vi "Run (WaveIO).vi"(8 "error in (no error)":errorcluster, 11 "Audio Output Queue":refnum<queue>) -> (0 "error out":errorcluster)   [LabVIEW 2018, in "Audio Output.lvlib"]
doc: "The main audio output loop.\n\n<b>Priority:</b> Time Critical\n<b>Execution System:</b> Instrument I/O"
uses:
  Audio Output.lvlib
  Audio Output Queue Type.ctl
  State.ctl
  Messaging/Message Cluster.ctl
  Audio Output Config.ctl
  Audio Output Info.ctl
  external/waveio_108/WaveIO.llb/SoundHandle.ctl
  Globals/Debug.vi
  Messaging/Messaging.lvlib
  <vilib>/ptbypt/NI_PtbyPt.lvlib
  Globals/Globals.lvlib
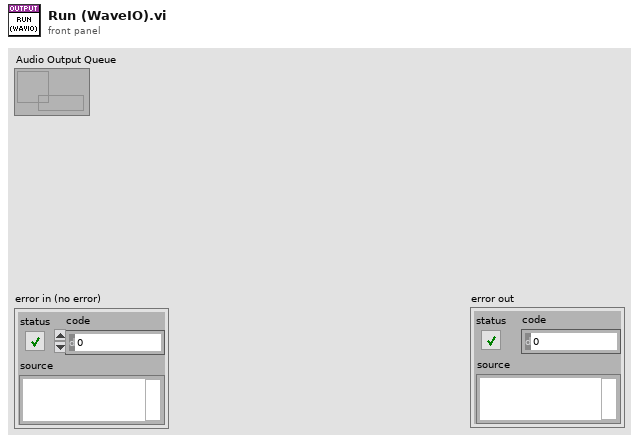
[diagram p1: front panel]
types:
  T1 = typedef "Audio Output.lvlib/Audio Output Config.ctl" = cluster{"Master":T2, "Headphones":T2}
  T2 = typedef "Audio Output.lvlib/Audio Output Info.ctl" = cluster{"Enable":bool, "Output ID":i32}
  T3 = typedef "Messaging.lvlib/Message Cluster.ctl" = cluster{"Event":string, "Source":string, "Target":string, "Data":variant}
  T4 = typedef "Audio Output.lvlib/State.ctl" = enum16{"Init", "Configure", "Output", "Error", "Shutdown"}
  T5 = typedef "SoundHandle.ctl" = cluster{"DeviceID":u16, "Samples/buf":u32, "Sampl rate":u32, "Bits/sample":u16, "Channels":u8, "Opened":bool}
  T6 = cluster{"# buffers":i32, "Buffer size":i32, "unit (ms)":enum16{"time (ms)", "Samples"}}
  T7 = typedef "Audio Output.lvlib/Audio Output Queue Type.ctl" = cluster{"Master":waveform(i16)[], "Headphones":waveform(i16)[], "Start Time":dbl}
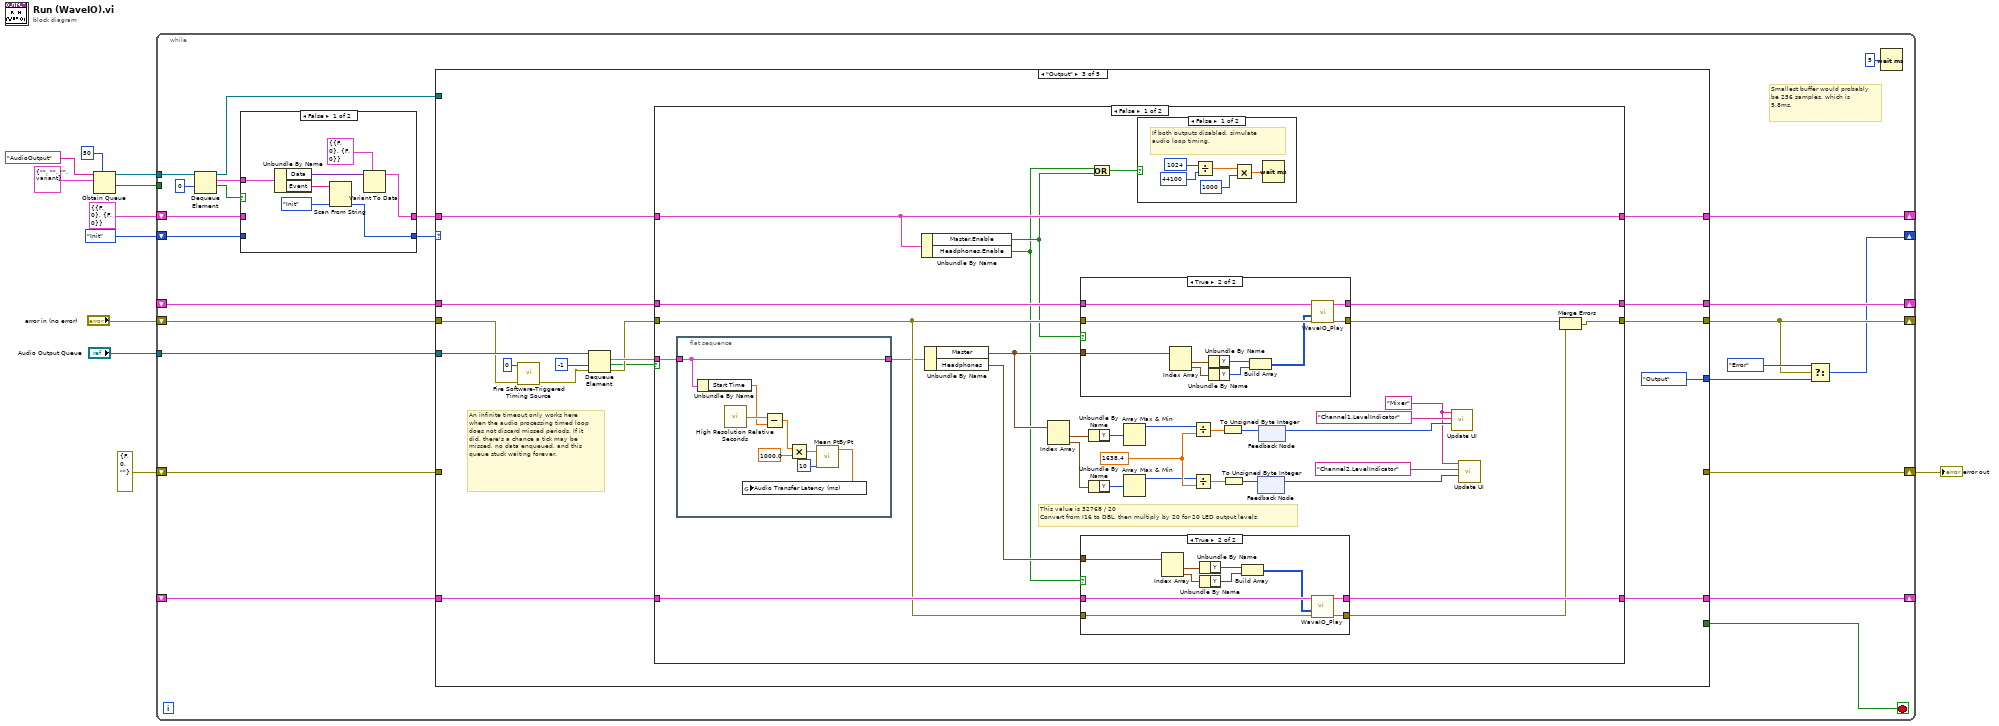
[diagram p0: block diagram]
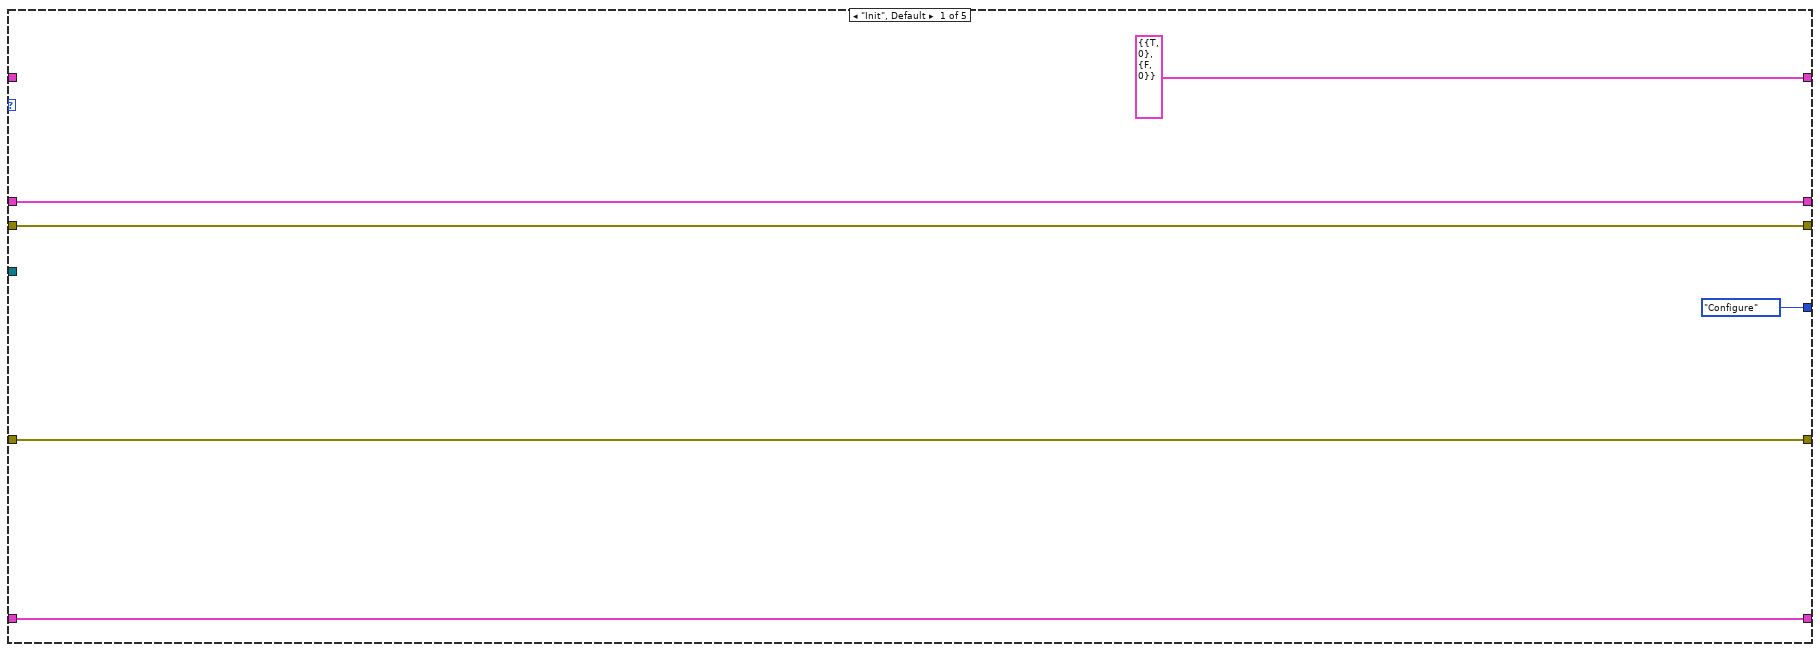
[diagram p3: hidden frame]
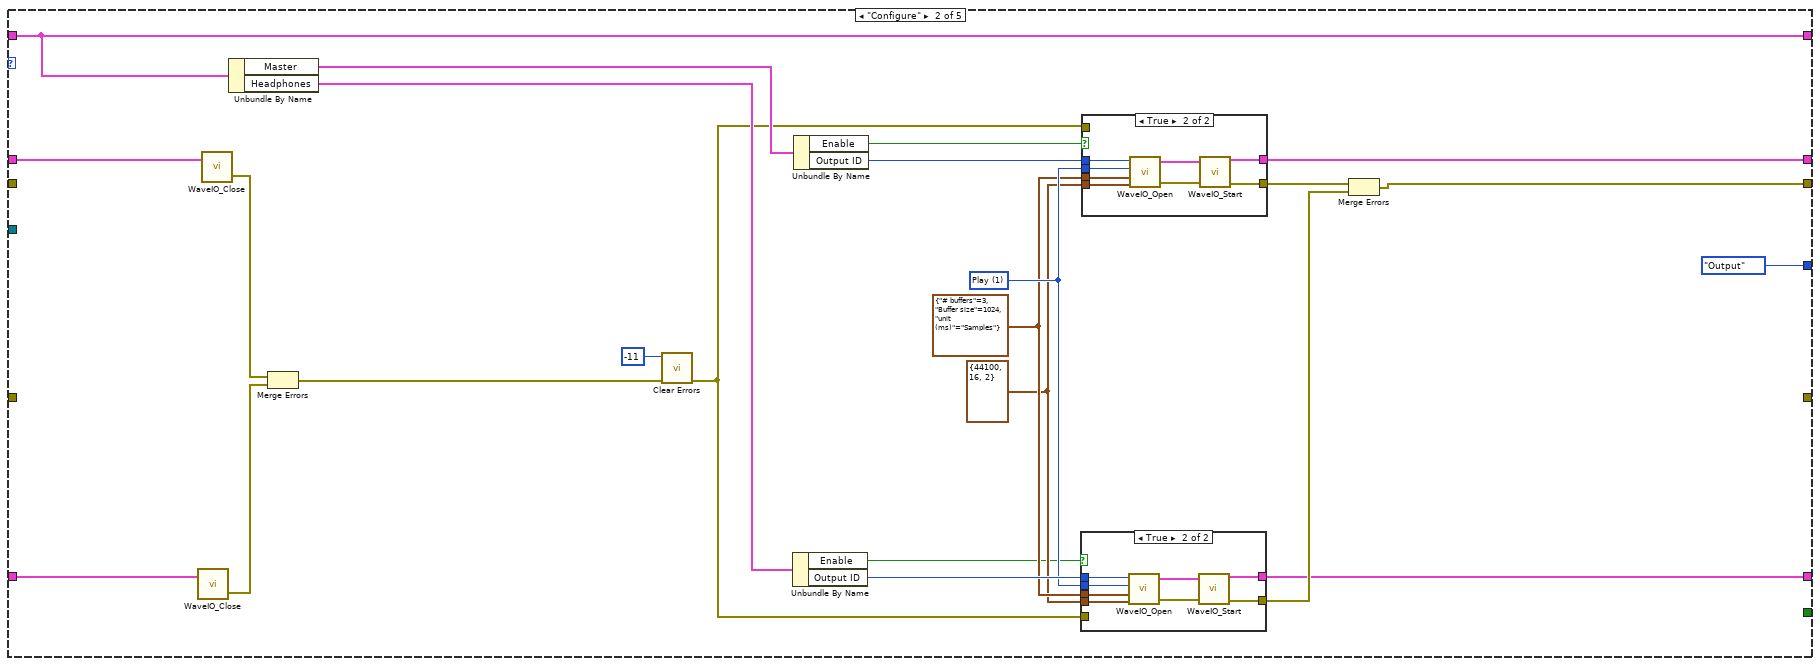
[diagram p4: hidden frame]
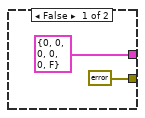
[diagram p5: hidden frame]
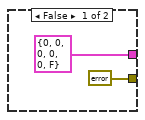
[diagram p6: hidden frame]
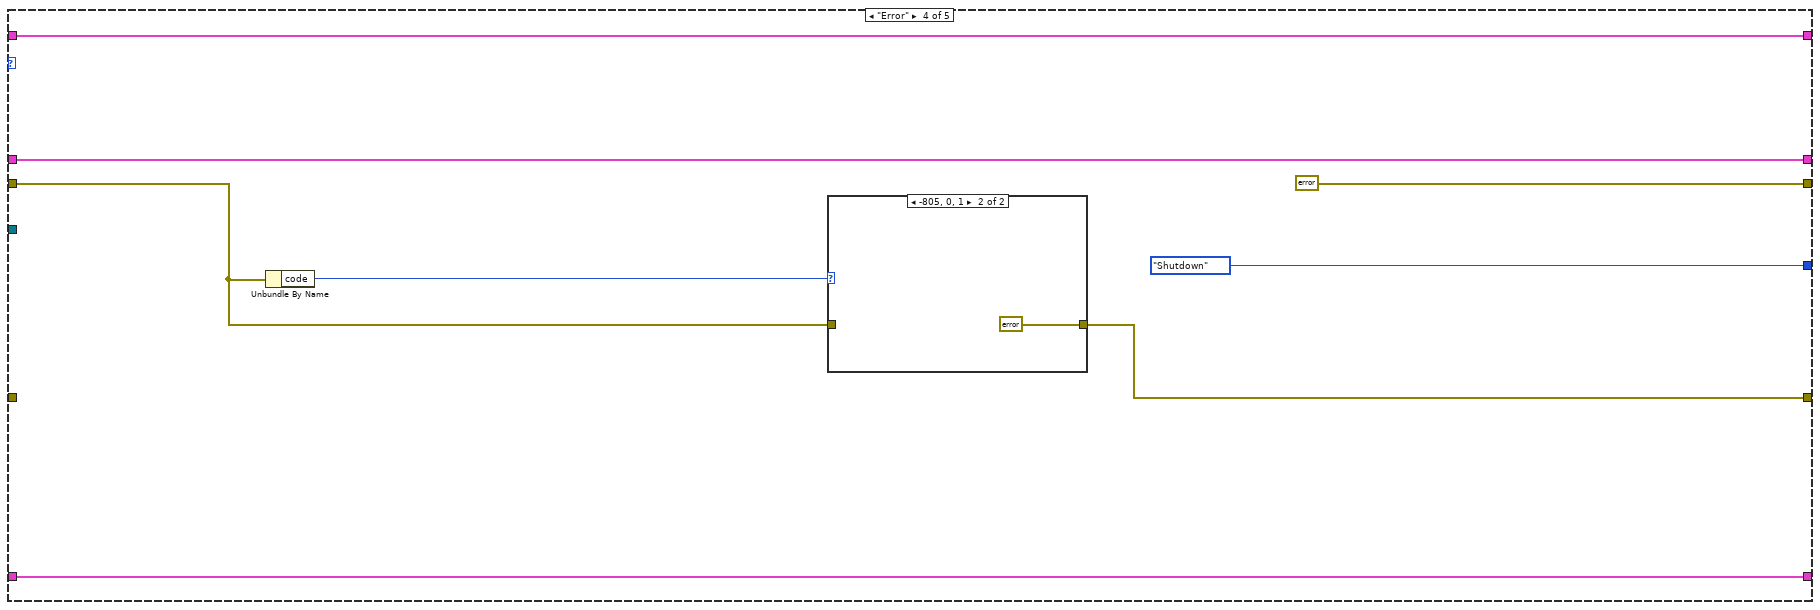
[diagram p11: hidden frame]
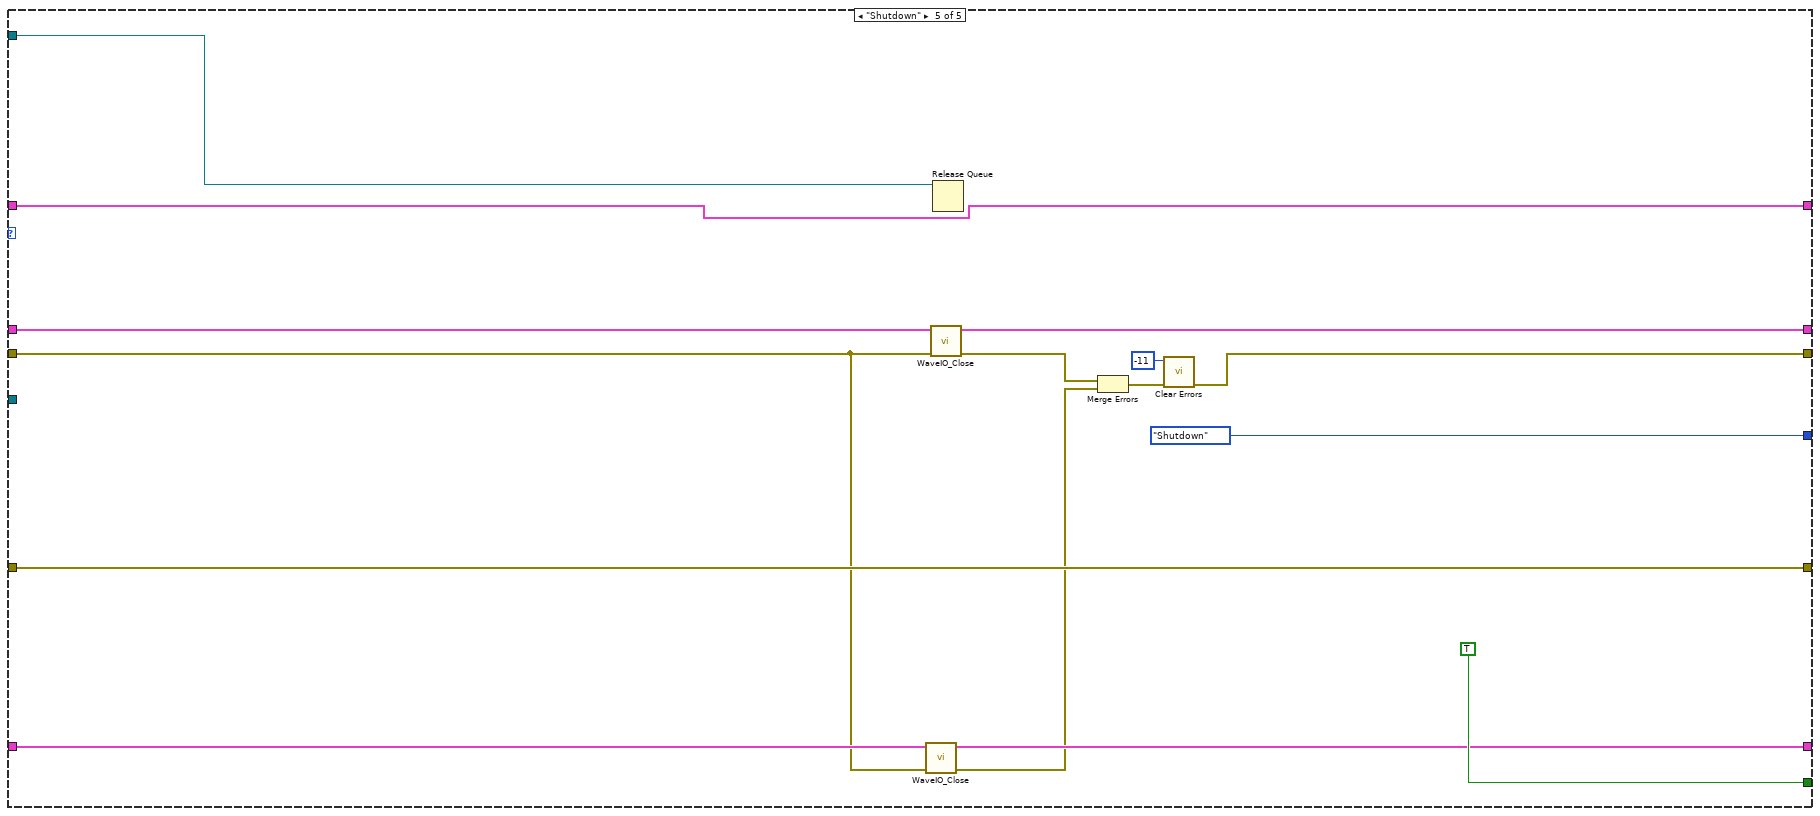
[diagram p13: hidden frame]
diagram:
  n1 = Obtain Queue(max queue size (-1, unlimited)=50, name (unnamed)="AudioOutput", element data type=T3 {"Event"="", "Source"="", "Target"="", "Data"=variant} ("Message")) -> (queue out=w4:refnum<queue>, created new?=w3:bool)  [unwired: 2 in, 1 out]
  n2 = while {
    shift-right: [w30] -> _
    shift-left: State."Init" ("State") -> [w19]
    shift-right: [w35] -> _
    shift-left: _ -> [w34]
    shift-right: [w31] -> _
    shift-left: "error in (no error)" -> [w29]
    tunnel: "Audio Output Queue" -> [w27]
    shift-right: [w26] -> w9
    shift-left: errorcluster {"status"=FALSE, "code"=0, "source"=""} ("error out") -> [w25]
    shift-right: [w24] -> _
    shift-left: _ -> [w23]
    tunnel: w4 -> [w21]
    shift-right: [w13] -> _
    shift-left: T1 {"Master"={"Enable"=FALSE, "Output ID"=0}, "Headphones"={"Enable"=FALSE, "Output ID"=0}} -> [w15]
    tunnel: w3 -> [_]
    stop <- w28 stop-if-true
    # "Smallest buffer would probably be 256 samples, which is 5.8ms."
    n3 = Dequeue Element(queue=w21, timeout in ms (-1)=0) -> (queue out=w16:refnum<queue>, element=w20:T3, timed out?=w17:bool)  [unwired: 1 in, 1 out]
    n4 = case shown="False" w17 {
      tunnel: w20 -> [w42 _]
      tunnel: w19 -> [_ w44]
      tunnel: [w39 w44] -> w18
      tunnel: [w36 w43] -> w14
      tunnel: w15 -> [_ w43]
      frame False {
        n5 = Unbundle By Name(w42) -> ("Data"=w37:variant, "Event"=w41:string)
        n6 = Scan From String(input string=w41, default 1=State."Init" ("State")) -> (output 1=w39:T4)  [unwired: 3 in, 3 out]
        n7 = Variant To Data(type=T1 {"Master"={"Enable"=FALSE, "Output ID"=0}, "Headphones"={"Enable"=FALSE, "Output ID"=0}}, Variant=w37) -> (data=w36:T1)  [unwired: 1 in, 1 out]
      }
      frame True {
      }
    }
    n8 = case shown="\"Output\"" w18 {
      tunnel: [w49 w73 w107 w190 w206] -> w35
      tunnel: w34 -> [w49 w69 w109 w190 w207]
      tunnel: [w48 w70 w108 errorcluster {"status"=FALSE, "code"=0, "source"=""} ("error out") w194] -> w31
      tunnel: [State."Configure" ("State") State."Output" ("State") State."Output" ("State") State."Shutdown" ("State") State."Shutdown" ("State")] -> w33
      tunnel: w29 -> [w48 _ w94 w186 w198]
      tunnel: [_ _ _ _ TRUE] -> w28
      tunnel: w27 -> [_ _ w103 _ _]
      tunnel: [w47 _ _ w185 w203] -> w26
      tunnel: w25 -> [w47 _ _ _ w203]
      tunnel: [w46 w57 w100 w184 w201] -> w24
      tunnel: w23 -> [w46 w68 w99 w184 w202]
      tunnel: w16 -> [_ _ _ _ w200]
      tunnel: w14 -> [_ w63 w97 w183 w199]
      tunnel: [T1 {"Master"={"Enable"=TRUE, "Output ID"=0}, "Headphones"={"Enable"=FALSE, "Output ID"=0}} ("Audio Output Config") w63 w98 w183 w199] -> w13
      frame "Init", Default {
      }
      frame "Configure" {
        w59 = cluster{"Rate":i32, "Bits":i32, "Channels":u32} {"Rate"=44100, "Bits"=16, "Channels"=2} ("Format (44kHz, 16Bit, stereo)")
        w60 = T6 {"# buffers"=3, "Buffer size"=1024, "unit (ms)"=enum."Samples"} ("Buffer Config")
        w61 = u16 1 items=["Record", "Play", "Loopback", "ASIO input", "ASIO output", "Record (WASAPI)", "Play (WASAPI)", "Record Combi", "Play Combi"] ("device type (Record)")
        n9 = call "WaveIO_Close.vi"("Handle"=w68) -> ("error out"=w55:errorcluster)  [unwired: 1 in, 1 out]
        n10 = call "WaveIO_Close.vi"("Handle"=w69) -> ("error out"=w56:errorcluster)  [unwired: 1 in, 1 out]
        n11 = Unbundle By Name(w63) -> ("Master"=w67:T2, "Headphones"=w64:T2)
        n12 = Merge Errors(w56, w55) -> (w54:errorcluster)
        n13 = call <vilib>:"Clear Errors.vi"("error in (no error)"=w54, "specific error code to clear (0: all)"=-11) -> ("error out"=w53:errorcluster)  [unwired: 4 in, 1 out]
        n14 = Unbundle By Name(w64) -> ("Enable"=w51:bool, "Output ID"=w62:i32)
        n15 = Unbundle By Name(w67) -> ("Enable"=w52:bool, "Output ID"=w65:i32)
        n16 = case shown="True" w51 {
          tunnel: [T5 {"DeviceID"=0, "Samples/buf"=0, "Sampl rate"=0, "Bits/sample"=0, "Channels"=0, "Opened"=FALSE} ("Handle Out") w81] -> w57
          tunnel: [errorcluster {"status"=FALSE, "code"=0, "source"=""} ("error out") w80] -> w58
          tunnel: w61 -> [_ w79]
          tunnel: w60 -> [_ w78]
          tunnel: w59 -> [_ w77]
          tunnel: w62 -> [_ w76]
          tunnel: w53 -> [_ _]
          frame False {
          }
          frame True {
            n17 = call "WaveIO_Open.vi"("idev"=w76, "device type (Record)"=w79, "Buffer Config"=w78, "Format (44kHz, 16Bit, stereo)"=w77) -> ("Sound Handle Out"=w82:T5, "error out"=w83:errorcluster)  [unwired: 3 in]
            n18 = call "WaveIO_Start.vi"("error in (no error)"=w83, "Handle"=w82) -> ("error out"=w80:errorcluster, "Handle Out"=w81:T5)
          }
        }
        n19 = case shown="True" w52 {
          tunnel: [T5 {"DeviceID"=0, "Samples/buf"=0, "Sampl rate"=0, "Bits/sample"=0, "Channels"=0, "Opened"=FALSE} ("Handle Out") w91] -> w73
          tunnel: [errorcluster {"status"=FALSE, "code"=0, "source"=""} ("error out") w90] -> w71
          tunnel: w61 -> [_ w89]
          tunnel: w60 -> [_ w88]
          tunnel: w59 -> [_ w87]
          tunnel: w65 -> [_ w86]
          tunnel: w53 -> [_ _]
          frame False {
          }
          frame True {
            n20 = call "WaveIO_Open.vi"("idev"=w86, "device type (Record)"=w89, "Buffer Config"=w88, "Format (44kHz, 16Bit, stereo)"=w87) -> ("Sound Handle Out"=w92:T5, "error out"=w93:errorcluster)  [unwired: 3 in]
            n21 = call "WaveIO_Start.vi"("error in (no error)"=w93, "Handle"=w92) -> ("error out"=w90:errorcluster, "Handle Out"=w91:T5)
          }
        }
        n22 = Merge Errors(w71, w58) -> (w70:errorcluster)
      }
      frame "Output" {
        # "An infinite timeout only works here when the audio processing timed loop does not discard missed periods. If it did, there's a chance a tick may be missed, no data enqueued, and this queue stuck waiting forever."
        n23 = call <vilib>:"Fire Software-Triggered Timing Source.vi"("error in (no error)"=w94, "trigger ID"=u8 0) -> ("error out"=w95:errorcluster)  [unwired: 8 in, 1 out]
        n24 = Dequeue Element(queue=w103, timeout in ms (-1)=-1, error in (no error)=w95) -> (element=w105:T7, timed out?=w101:bool, error out=w102:errorcluster)  [unwired: 1 out]
        n25 = case shown="False" w101 {
          tunnel: w109 -> [w130 w182]
          tunnel: [w124 w181] -> w108
          tunnel: [w129 w182] -> w107
          tunnel: w105 -> [w111 _]
          tunnel: w102 -> [w120 w181]
          tunnel: [w128 w180] -> w100
          tunnel: w99 -> [w127 w180]
          tunnel: [w121 w179] -> w98
          tunnel: w97 -> [w121 w179]
          frame False {
            w114 = "Mixer" ("Target")
            w137 = 1638.4
            # "This value is 32768 / 20\nConvert from I16 to DBL, then multiply by 20 for 20 LED output levels"
            n26 = flat-sequence {
              tunnel: w111 -> [w149]
              tunnel: [w149] -> w110
              frame #0 {
                n27 = Unbundle By Name(w149) -> ("Start Time"=w147:dbl)
                n28 = call <vilib>:"High Resolution Relative Seconds.vi"() -> ("relative seconds"=w148:dbl)
                n29 = Subtract(x=w148, y=w147) -> (x-y=w146:dbl)
                n30 = Multiply(x=w146, y=1000.0) -> (x*y=w144:dbl)
                n31 = call <vilib>:"Mean PtByPt.vi"("x"=w144, "sample length"=10) -> ("mean"=w143:dbl)  [unwired: 2 in, 1 out]
                n32 = global write "Debug.vi" "Audio Transfer Latency (ms)"(w143) -> ()
              }
            }
            n33 = Unbundle By Name(w121) -> ("Master.Enable"=w119:bool, "Headphones.Enable"=w118:bool)
            n34 = Unbundle By Name(w110) -> ("Master"=w123:waveform(i16)[], "Headphones"=w122:waveform(i16)[])
            n35 = Index Array(array=w123) -> (element #1=w132:waveform(i16), element #2=w133:waveform(i16))  [unwired: 2 in]
            n36 = case shown="True" w119 {
              tunnel: w130 -> [w168 w174]
              tunnel: [w168 w173] -> w129
              tunnel: w120 -> [w167 w172]
              tunnel: [w167 w170] -> w125
              tunnel: w123 -> [_ w169]
              frame False {
              }
              frame True {
                n37 = Index Array(array=w169) -> (element #1=w175:waveform(i16), element #2=w176:waveform(i16))  [unwired: 2 in]
                n38 = Unbundle By Name(w175) -> ("Y"=w178:i16[])
                n39 = Unbundle By Name(w176) -> ("Y"=w177:i16[])
                n40 = Build Array(w178, w177) -> (w171:i16[][])
                n41 = call "WaveIO_Play.vi"("error in (no error)"=w172, "data"=w171, "Handle"=w174) -> ("error out"=w170:errorcluster, "Handle Out"=w173:T5)  [unwired: 1 in]
              }
            }
            n42 = case shown="True" w118 {
              tunnel: [w156 w166] -> w128
              tunnel: w127 -> [w156 w165]
              tunnel: [w155 w164] -> w126
              tunnel: w122 -> [_ w157]
              tunnel: w120 -> [w155 w158]
              frame False {
              }
              frame True {
                n43 = Index Array(array=w157) -> (element #1=w163:waveform(i16), element #2=w162:waveform(i16))  [unwired: 2 in]
                n44 = Unbundle By Name(w163) -> ("Y"=w160:i16[])
                n45 = Unbundle By Name(w162) -> ("Y"=w161:i16[])
                n46 = Build Array(w160, w161) -> (w159:i16[][])
                n47 = call "WaveIO_Play.vi"("error in (no error)"=w158, "data"=w159, "Handle"=w165) -> ("error out"=w164:errorcluster, "Handle Out"=w166:T5)  [unwired: 1 in]
              }
            }
            n48 = Unbundle By Name(w132) -> ("Y"=w131:i16[])
            n49 = Unbundle By Name(w133) -> ("Y"=w134:i16[])
            n50 = Or(x=w118, y=w119) -> (x .or. y?=w117:bool)
            n51 = Array Max & Min(array=w131) -> (max value=w135:i16)  [unwired: 3 out]
            n52 = Array Max & Min(array=w134) -> (max value=w136:i16)  [unwired: 3 out]
            n53 = case shown="False" w117 {
              frame False {
                # "If both outputs disabled, simulate audio loop timing."
                n54 = Divide(x=1024, y=44100) -> (x/y=w151:dbl)
                n55 = Multiply(x=w151, y=1000) -> (x*y=w150:dbl)
                n56 = Wait (ms)(milliseconds to wait=w150) -> ()  [unwired: 1 out]
              }
              frame True {
              }
            }
            n57 = Divide(x=w135, y=w137) -> (x/y=w138:dbl)
            n58 = Divide(x=w136, y=w137) -> (x/y=w139:dbl)
            n59 = To Unsigned Byte Integer(number=w138) -> (unsigned 8bit integer=w140:u8)
            n60 = To Unsigned Byte Integer(number=w139) -> (unsigned 8bit integer=w141:u8)
            n61 = feedback #1() -> (w112:u8)  [unwired: 1 in]
            n62 = feedback-in #1(w141) -> ()
            n63 = feedback #2() -> (w115:u8)  [unwired: 1 in]
            n64 = feedback-in #2(w140) -> ()
            n65 = call "Update UI.vi"("Data"=w115, "Target"="Channel1.LevelIndicator", "ID"=w114) -> ()  [unwired: 8 in, 1 out]
            n66 = call "Update UI.vi"("Data"=w112, "Target"="Channel2.LevelIndicator", "ID"=w114) -> ()  [unwired: 8 in, 1 out]
            n67 = Merge Errors(w125, w126) -> (w124:errorcluster)
          }
          frame True {
          }
        }
      }
      frame "Error" {
        n68 = Unbundle By Name(w186) -> ("code"=w187:i32)
        n69 = case shown="-805, 0, 1" w187 {
          tunnel: w186 -> [w191 _]
          tunnel: [w191 errorcluster {"status"=FALSE, "code"=0, "source"=""} ("error out")] -> w185
          frame Default {
          }
          frame -805, 0, 1 {
          }
        }
      }
      frame "Shutdown" {
        n70 = call "WaveIO_Close.vi"("error in (no error)"=w198, "Handle"=w202) -> ("error out"=w196:errorcluster, "Handle Out"=w201:T5)
        n71 = call "WaveIO_Close.vi"("error in (no error)"=w198, "Handle"=w207) -> ("error out"=w197:errorcluster, "Handle Out"=w206:T5)
        n72 = Release Queue(queue=w200) -> ()  [unwired: 2 in, 3 out]
        n73 = Merge Errors(w197, w196) -> (w195:errorcluster)
        n74 = call <vilib>:"Clear Errors.vi"("error in (no error)"=w195, "specific error code to clear (0: all)"=-11) -> ("error out"=w194:errorcluster)  [unwired: 4 in, 1 out]
      }
    }
    n75 = Select(t=State."Error" ("State"), s=w31, f=w33) -> (s? t:f=w30:T4)
    n76 = Wait (ms)(milliseconds to wait=u32 5 ("millisecond multiple")) -> ()  [unwired: 1 out]
  }
  "error out" <- w9
